vi "Dashboard Main.vi"() -> ()   [LabVIEW 2012]
uses:
  <vilib>/Utility/config.llb/Read Key (String).vi
  <vilib>/Utility/config.llb/Read Key (I32).vi
  <vilib>/Utility/config.llb/Write Key (String).vi
  <vilib>/Utility/config.llb/Write Key (I32).vi
  <vilib>/Utility/config.llb/NI_LVConfig.lvlib
panel:
  in  "Enable 4":bool
  in  "Camera Settings 2":T1={"Frate Rate"=30, "Compression"=30, "Size"=1} {"Frate Rate" scale=1.0..30.0; "Size" items=["640x480", "320x240", "160x120"]}
  in  "Enable 3":bool
  out "Mbps 3":dbl format="%#.1g"
  in  "Enable 2":bool
  in  "DB Camera Config 2":bool
  out "Mbps 2":bool
  out "fps 2":dbl format="%#.1g"
  out "Camera Image 2":T2(plugin-control)
  out "Battery Value":dbl(slide) scale=0.0..14.0 scale format="%#_2e"
  out "Battery":sgl(graph)
  in  "Camera Settings":T1={"Frate Rate"=30, "Compression"=30, "Size"=1} {"Frate Rate" scale=1.0..30.0; "Size" items=["640x480", "320x240", "160x120"]}
  out "Mode":T3(ring)=enum."Auto Disabled"
  out "JS1 Z":dbl(slide) scale=-1.0..1.0 scale format="%#_2e"
  out "JS2 Z":dbl(slide) scale=-1.0..1.0 scale format="%#_2e"
  out "Joystick 1":cluster{"X":dbl, "Y":dbl}[](graph)
  out "Joystick 2":cluster{"X":dbl, "Y":dbl}[](graph)
  out "JS Buttons 1":T4
  out "JS Buttons 2":T4
  out "MotorSlide4":dbl(slide) scale=-1.0..1.0 scale format="%#_2e"
  out "MotorSlide3":dbl(slide) scale=-1.0..1.0 scale format="%#_2e"
  out "MotorSlide2":dbl(slide) scale=-1.0..1.0 scale format="%#_2e"
  in  "MotorName3":string="Front Left"
  in  "MotorName4":string="Front Right"
  in  "MotorName1":string="Rear Left"
  in  "MotorName2":string="Rear Right"
  out "MotorChart4":dbl(graph)
  out "MotorChart3":dbl(graph)
  out "MotorChart2":dbl(graph)
  out "MotorSlide1":dbl(slide) scale=-1.0..1.0 scale format="%#_2e"
  out "MotorChart1":dbl(graph)
  out "Robot IP":string
  in  "Dashboard Tab":enum32{"Controls", "Test"}(tab)
  out "Climb Mode":bool
  out "Shooter Ready":bool
  out "Driver Ready":bool
  out "Manual Mode":bool
  in  "Slider":dbl(slide) scale=0.0..100.0 scale format="%#_3g"
  in  "On/Off":bool caption="Solenoid"
  in  "Test Name":u16(ring) items=["Select the test to run...", "Example Test", "-------------------------------", "List of tests is built in robot code.", "Replace with your own automated tests."]
  in  "Test Tree":string(tree)
  in  "Motor":cluster{"Value":dbl, "Enable":bool} {"Value" scale=-1.0..1.0 scale format="%#_3g"}
  out "Progress":T5 {"Test Progress" scale=0.0..100.0}
  in  "Rev/Fwd":cluster{"Forward":bool, "Reverse":bool}
  in  "Ring":u16(ring) items=["Auto", "Fixed indoor", "Fixed outdoor 1", "Fixed outdoor 2", "Fixed fluorescent 1", "Fixed fluorescent 2", "Hold current"]
  in  "Viewer":enum32{"Camera Image", "Variables"}(tab)
  out "Mbps":dbl format="%#.1g"
  in  "Enable":bool
  in  "DB Camera Config":bool
  out "Mbps":bool
  out "fps":dbl format="%#.1g"
  out "Image Error Message":string="Timeout in Camera Communications"
  out "Camera Image":T2(plugin-control)
  out "Tree":string(tree)
  # "Drive & Motors"
  # "Robot IP:"
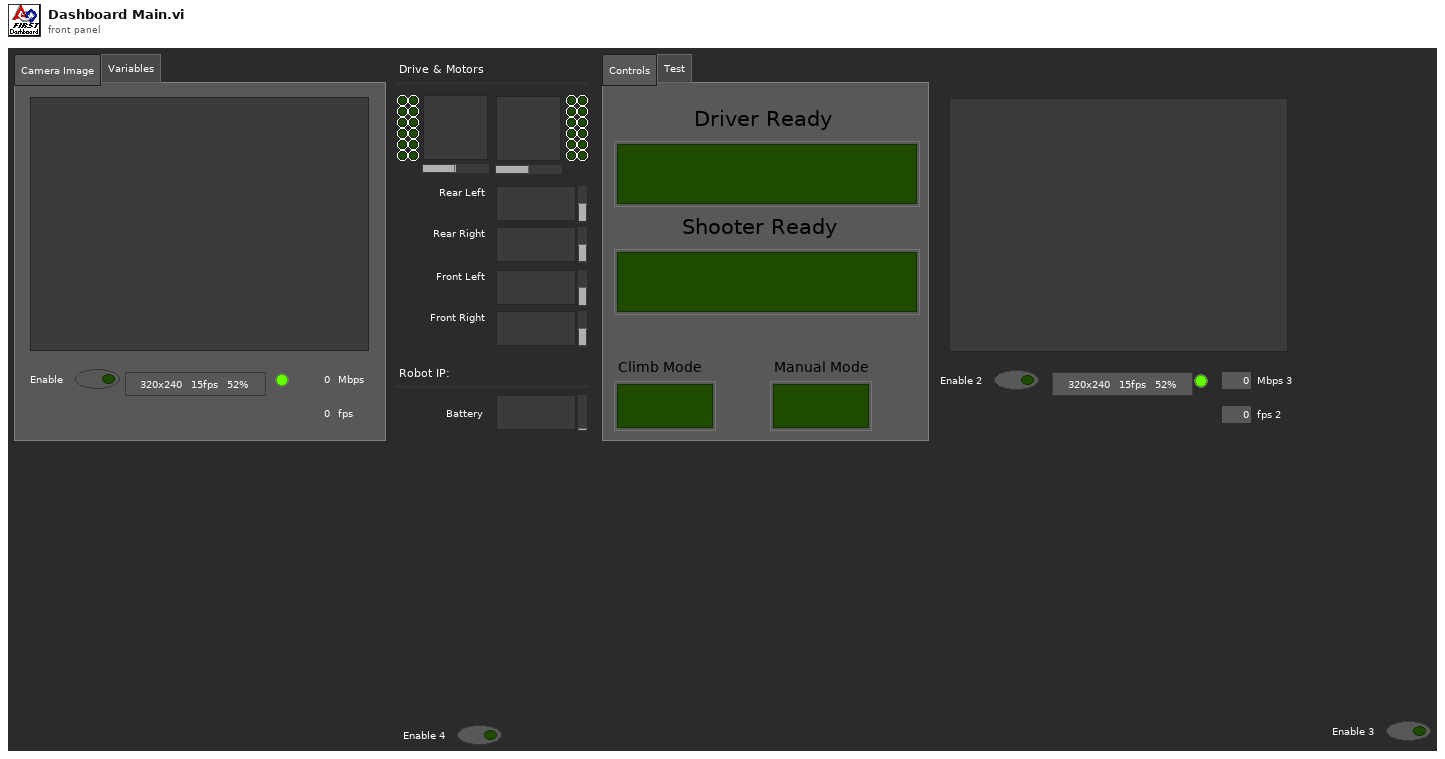
[diagram p1: front panel]
types:
  T1 = cluster{"Frate Rate":i32, "Compression":i32, "Size":u16}
  T2 = typedef "IMAQ Image.ctl" = refnum<image>
  T3 = enum8{"Tele-Op Disabled", "Tele-Op Enabled", "Auto Disabled", "Auto Enabled", "Test Disabled", "Test Enabled", ""}
  T4 = cluster{bool, bool, bool, bool, bool, bool, bool, bool, bool, bool, bool, bool}
  T5 = cluster{"Test Progress":u8, "Test Progress Text":string}
  T6 = typedef "Image Type" = u32
  T7 = typedef "NI_LVConfig.lvlib/Config Data RefNum.ctl" = refnum<k1>
  T8 = cluster{"Competition mode":bool, "Robot Link":bool, "Autonomous":bool, "Enabled":bool, "E-Stop":bool, "Simulated":bool, "TestMode":bool, "Docked Window":bool}
  T9 = cluster{"Boolean Array[0]":bool, "Boolean Array[1]":bool, "Boolean Array[2]":bool, "Boolean Array[3]":bool, "Boolean Array[4]":bool, "Boolean Array[5]":bool, "Boolean Array[6]":bool, "Boolean Array[7]":bool, "Boolean Array[8]":bool, "Boolean Array[9]":bool, "Boolean Array[10]":bool, "Boolean Array[11]":bool}
  T10 = typedef "LVRectTypeDef.ctl" = cluster{"Left":i16, "Top":i16, "Right":i16, "Bottom":i16}
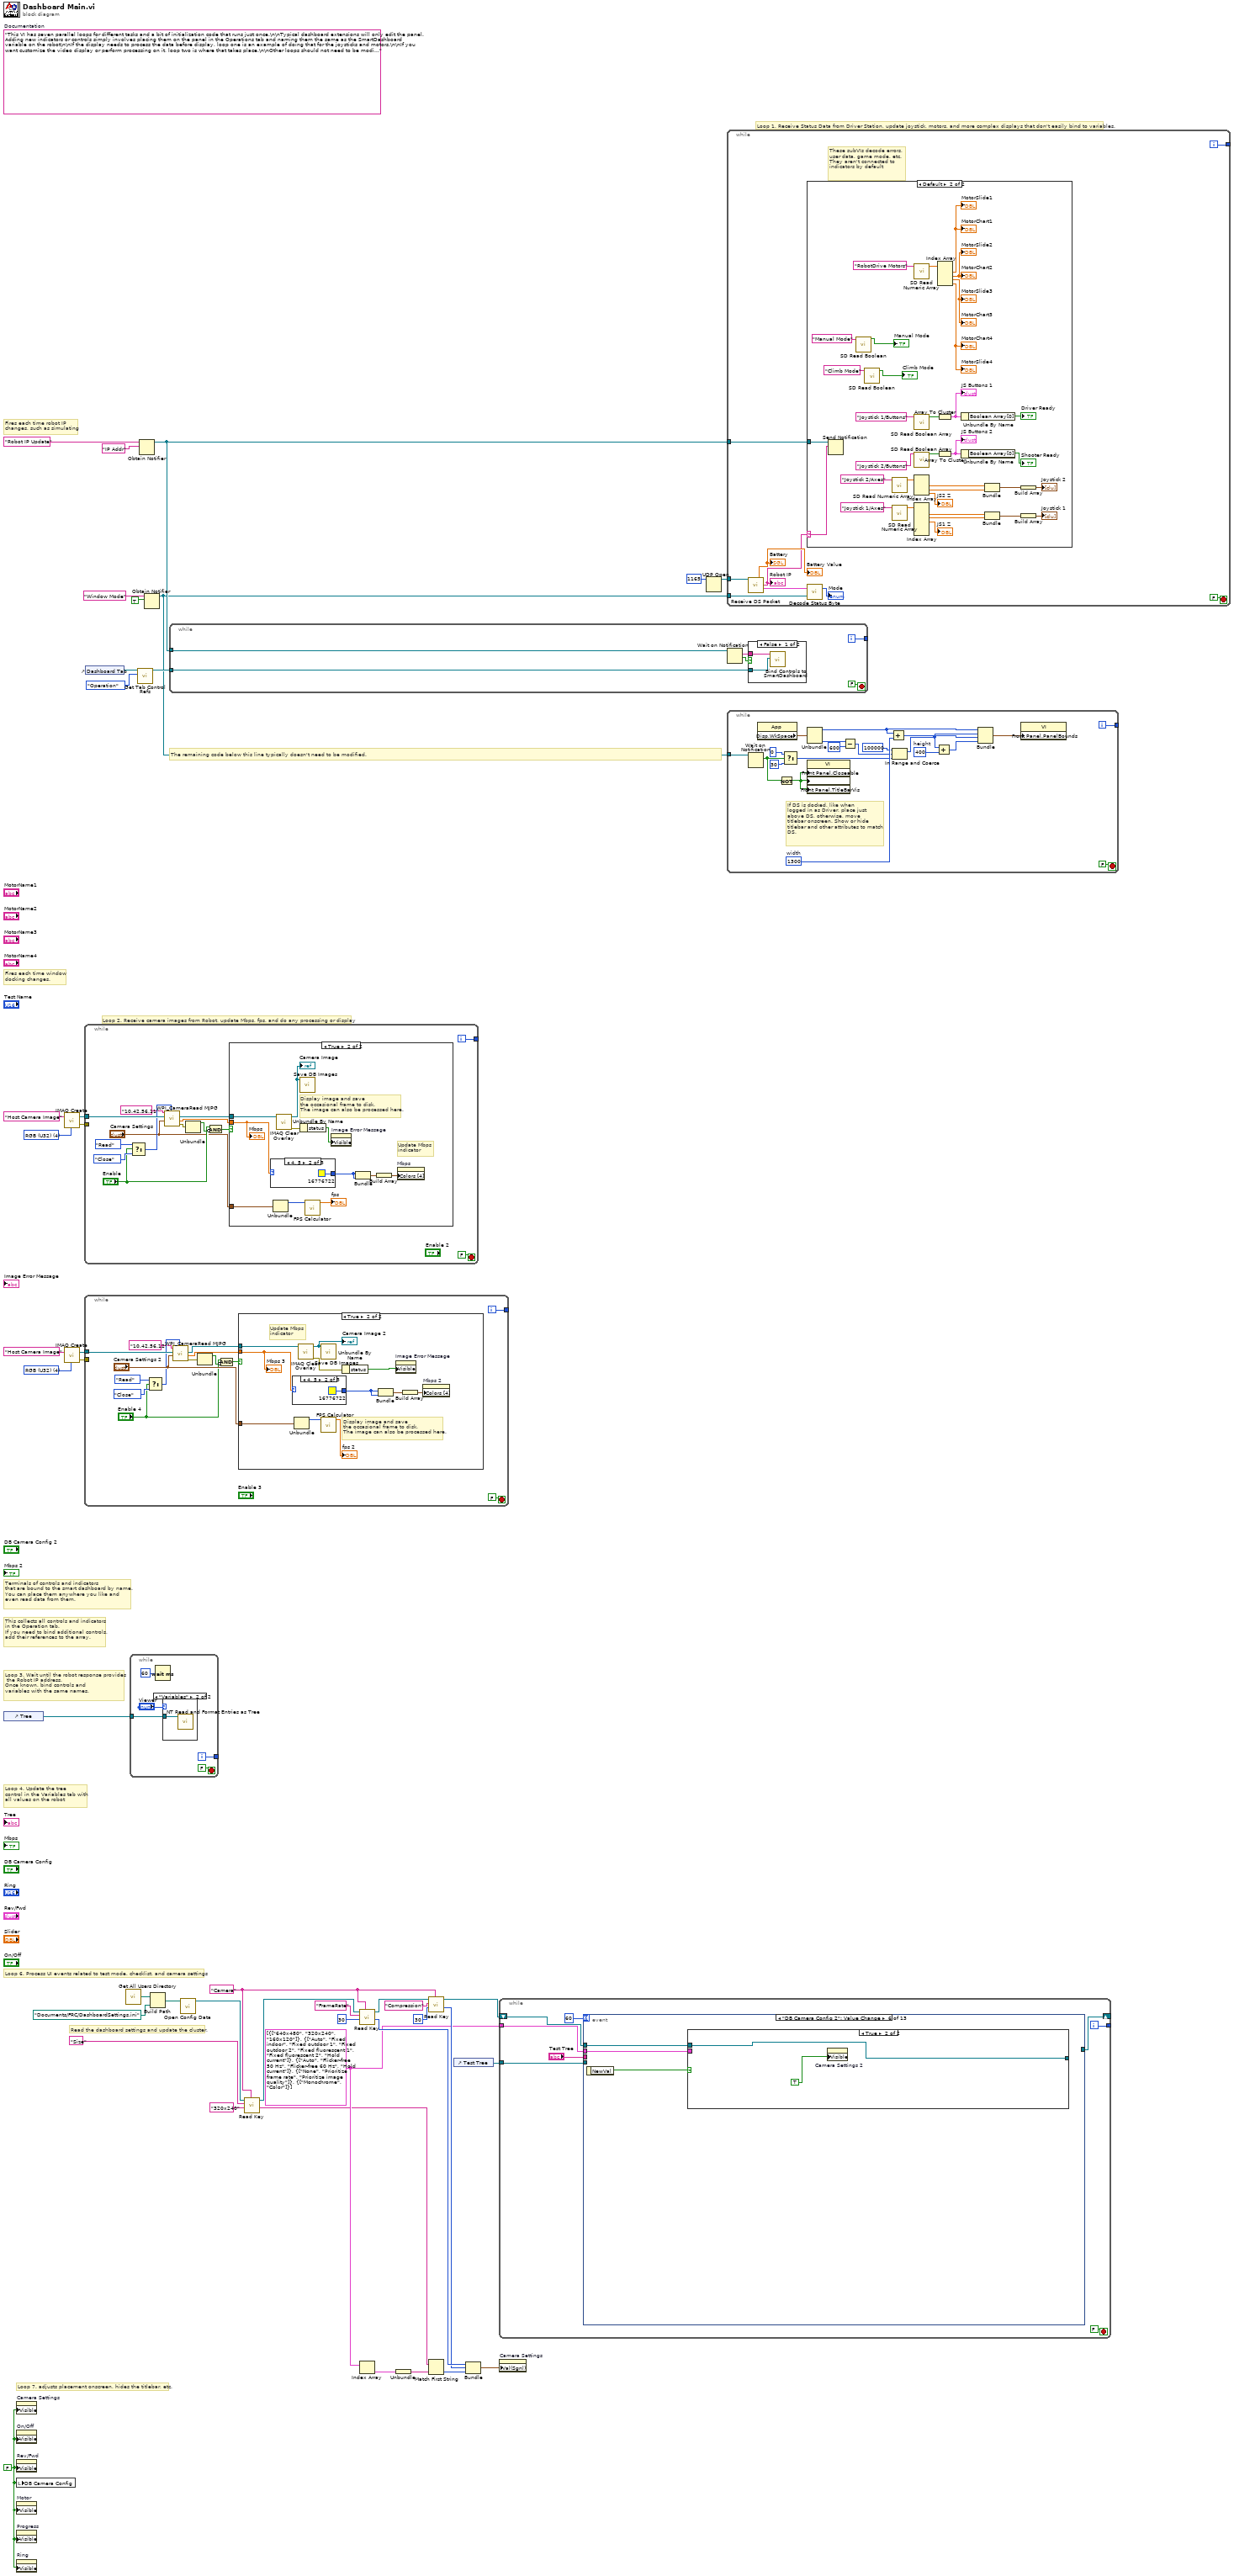
[diagram p0: block diagram]
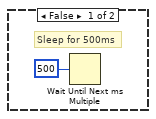
[diagram p2: hidden frame]
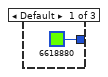
[diagram p3: hidden frame]
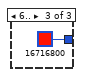
[diagram p4: hidden frame]
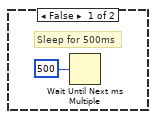
[diagram p6: hidden frame]
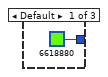
[diagram p7: hidden frame]
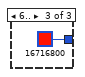
[diagram p8: hidden frame]
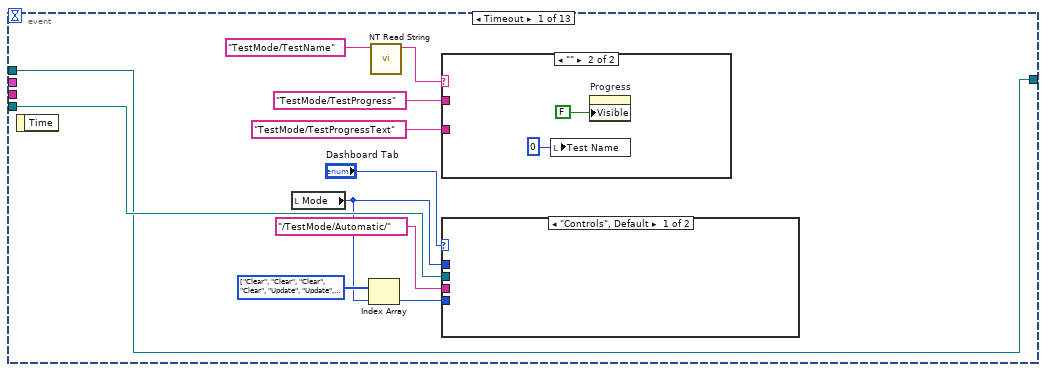
[diagram p9: hidden frame]
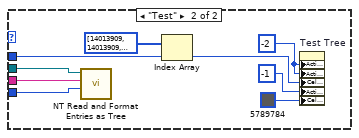
[diagram p10: hidden frame]
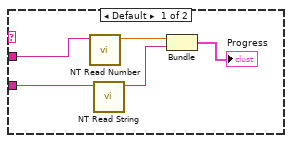
[diagram p11: hidden frame]
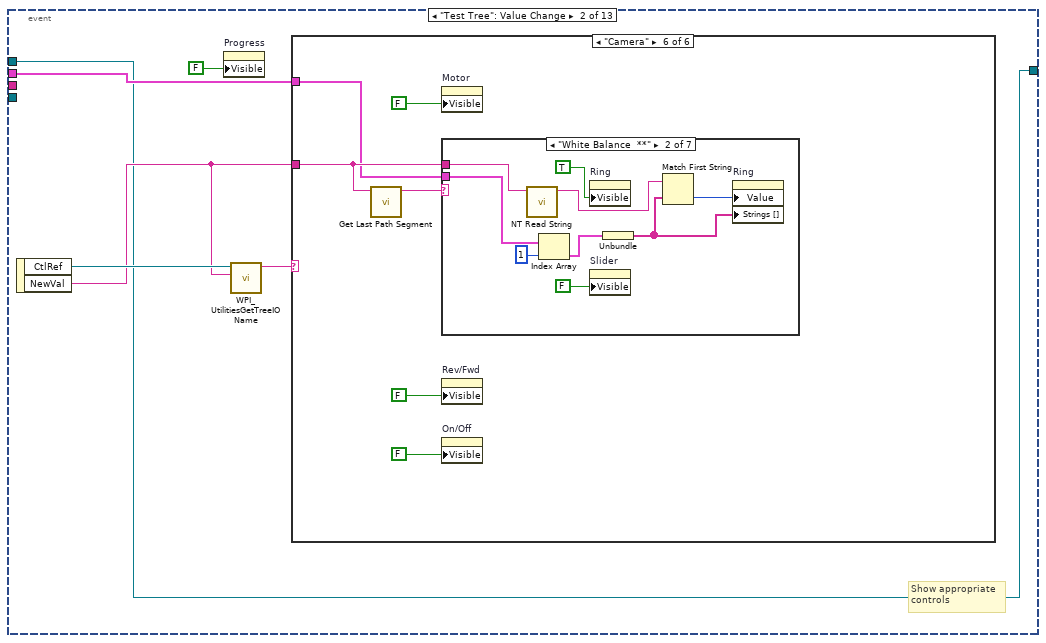
[diagram p12: hidden frame]
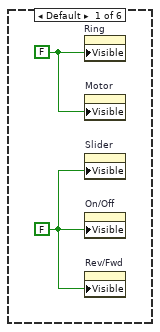
[diagram p13: hidden frame]
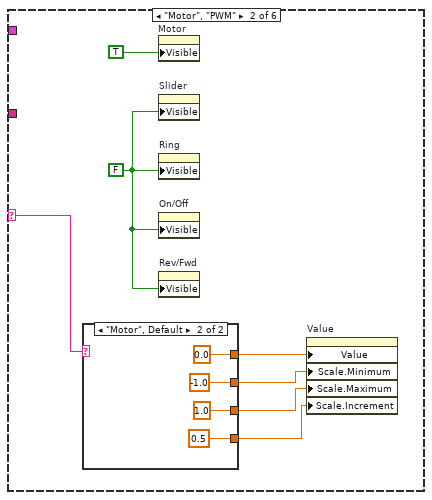
[diagram p14: hidden frame]
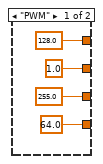
[diagram p15: hidden frame]
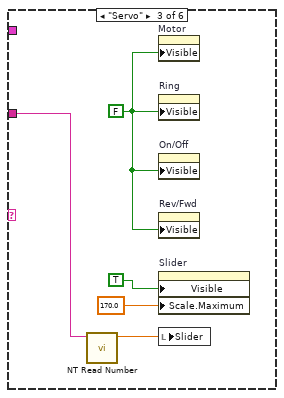
[diagram p16: hidden frame]
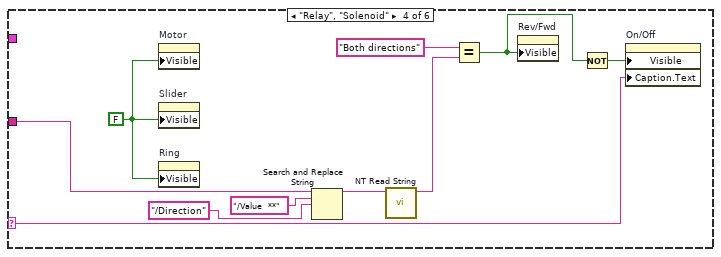
[diagram p17: hidden frame]
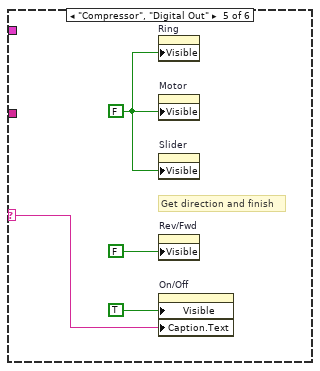
[diagram p18: hidden frame]
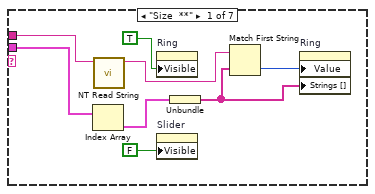
[diagram p19: hidden frame]
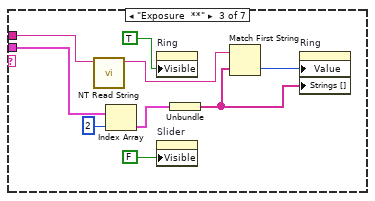
[diagram p20: hidden frame]
diagram:
  w4 = T6 4 items=["Grayscale (U8)", "Grayscale (I16)", "Grayscale (SGL)", "Complex (CSG)", "RGB (U32)", "HSL (U32)", "RGB (U64)"] ("Image Type")
  w23 = "Camera"
  w15 = cluster{string[]}[] [{["640x480", "320x240", "160x120"]}, {["Auto", "Fixed indoor", "Fixed outdoor 1", "Fixed outdoor 2", "Fixed fluorescent 1", "Fixed fluorescent 2", "Hold current"]}, {["Auto", "Flicker-free 50 Hz", "Flicker-free 60 Hz", "Hold current"]}, {["None", "Prioritize frame rate", "Prioritize image quality"]}, {["Monochrome", "Color"]}]
  w29 = FALSE ("Visible")
  (unwired) "This VI has seven parallel loops for different tasks and a bit of initialization code that runs just once.\n\nTypical dashboard extensions will only edit the panel. Adding new indicators or controls simply involves placing them on the panel in the Operations tab and naming them the same as the SmartDashboard variable on the robot\n\nIf the display needs to process the data before display, loop one is an example of doing that for the joysticks and motors.\n\nIf you want customize the video display or perform processing on it, loop two is where that takes place.\n\nOther loops should not need to be modified. They are pretty standard, and document the task they perform."  # Documentation
  w42 = T6 4 items=["Grayscale (U8)", "Grayscale (I16)", "Grayscale (SGL)", "Complex (CSG)", "RGB (U32)", "HSL (U32)", "RGB (U64)"] ("Image Type")
  # "Fires each time robot IP\nchanges, such as simulating"
  # "Fires each time window\ndocking changes."
  # "This collects all controls and indicators\nin the Operation tab.\nIf you need to bind additional controls,\nadd their references to the array."
  # "The remaining code below this line typically doesn't need to be modified."
  # "Loop 6. Process UI events related to test mode, checklist, and camera settings"
  # "Read the dashboard settings and update the cluster."
  # "Terminals of controls and indicators\nthat are bound to the smart dashboard by name.\nYou can place them anywhere you like and\neven read data from them."
  # "Loop 4. Update the tree\ncontrol in the Variables tab with\nall values on the robot"
  # "Loop 3. Wait until the robot response provides\n the Robot IP address.\nOnce known, bind controls and\nvariables with the same names."
  # "Loop 7. adjusts placement onscreen, hides the titlebar, etc."
  # "Loop 1. Receive Status Data from Driver Station, update joystick, motors, and more complex displays that don't easily bind to variables."
  # "Loop 2. Receive camera images from Robot, update Mbps, fps, and do any processing or display"
  n1 = control-ref of="Tree"() -> (w6:refnum<vi>)
  n2 = property on="Camera Settings" class="Clust (strict)"("Visible"=w29) -> ()  [unwired: 2 in, 2 out]
  n3 = property on="On/Off" class="Bool (strict)"("Visible"=w29) -> ()  [unwired: 2 in, 2 out]
  n4 = property on="Rev/Fwd" class="Clust (strict)"("Visible"=w29) -> ()  [unwired: 2 in, 2 out]
  n5 = local write "DB Camera Config"(w29) -> ()
  n6 = property on="Motor" class="Clust (strict)"("Visible"=w29) -> ()  [unwired: 2 in, 2 out]
  n7 = property on="Progress" class="Clust (strict)"("Visible"=w29) -> ()  [unwired: 2 in, 2 out]
  n8 = property on="Ring" class="Ring (strict)"("Visible"=w29) -> ()  [unwired: 2 in, 2 out]
  n9 = call "IMAQ Create"("Image Name"="Host Camera Image", "Image Type"=w42) -> ("New Image"=w40:T2, "error out"=w39:errorcluster)  [unwired: 2 in, 1 out]
  n10 = call "IMAQ Create"("Image Name"="Host Camera Image", "Image Type"=w4) -> ("New Image"=w2:T2, "error out"=w1:errorcluster)  [unwired: 2 in, 1 out]
  n11 = while {
    tunnel: w40 -> [w56]
    tunnel: w39 -> [_]
    tunnel: [w57] -> _
    i -> [w57]
    stop <- FALSE stop-if-true
    n12 = Select(t=enum16{"Read", "Reopen", "Close"}."Read" ("Operation"), s="Enable", f=enum16{"Read", "Reopen", "Close"}."Close" ("Operation")) -> (s? t:f=w51:enum16{"Read", "Reopen", "Close"})
    n13 = call <vilib>:"WPI_CameraRead MJPG.vi"("Operation"=w51, "Camera Settings"="Camera Settings", "Image"=w56, "address"="10.42.56.11") -> ("error out"=w50:errorcluster, "Bandwidth (kbps)"=w54:dbl, "Image Out"=w55:T2)  [unwired: 5 in]
    n14 = Unbundle(w50) -> ("status"=w48:bool)  [unwired: 2 out]
    n15 = Compound Arithmetic op=AND("Enable", invert w48) -> (w47:bool)
    n16 = case shown="True" w47 {
      tunnel: "Camera Settings" -> [_ w61]
      tunnel: w55 -> [_ w64]
      tunnel: w54 -> [_ w63]
      frame False {
        # "Sleep for 500ms"
        n17 = Wait Until Next ms Multiple(millisecond multiple=u32 500) -> ()  [unwired: 1 out]
      }
      frame True {
        # "Display image and save\nthe occasional frame to disk.\nThe image can also be processed here."
        # "Update Mbps\nindicator"
        n18 = case shown="4, 5" w63 {
          tunnel: [u32 6618880 ("Color Box") u32 16776722 ("Color Box") u32 16716800 ("Color Box")] -> w65
          frame Default {
          }
          frame 4, 5 {
          }
          frame 6.. {
          }
        }
        n19 = Unbundle(w61) -> ("Frate Rate"=w60:i32)  [unwired: 2 out]
        n20 = call "IMAQ Clear Overlay"("Image"=w64) -> ("error out"=w69:errorcluster, "Image Out"=w68:T2)  [unwired: 2 in, 7 out]
        "Camera Image" <- w68
        n21 = call "Save DB Images.vi"("Image"=w68) -> ()  [unwired: 2 in, 1 out]
        n22 = Unbundle By Name(w69) -> ("status"=w70:bool)
        n23 = call "FPS Calculator.vi"("Average Count"=w60) -> ("fps"=→"fps":dbl)  [unwired: 10 in]
        n24 = property on="Image Error Message" class="Str"("Visible"=w70) -> ()  [unwired: 2 in, 2 out]
        n25 = Bundle("Color Box"=w65, "Color Box"=w65) -> (w67:cluster{"Color Box":u32, "Color Box":u32})  [unwired: 1 out]
        n26 = Build Array(w67) -> (w66:cluster{"Color Box":u32, "Color Box":u32}[])
        n27 = property on="Mbps" class="Bool (strict)"("Colors [4]"=w66) -> ()  [unwired: 2 in, 2 out]
        "Mbps" <- w63
      }
    }
  }
  n28 = while {
    tunnel: w2 -> [w84]
    tunnel: w1 -> [_]
    tunnel: [w86] -> _
    i -> [w86]
    stop <- FALSE stop-if-true
    n29 = Select(t=enum16{"Read", "Reopen", "Close"}."Read" ("Operation"), s="Enable 4", f=enum16{"Read", "Reopen", "Close"}."Close" ("Operation")) -> (s? t:f=w79:enum16{"Read", "Reopen", "Close"})
    n30 = call <vilib>:"WPI_CameraRead MJPG.vi"("Operation"=w79, "Camera Settings"="Camera Settings 2", "Image"=w84, "address"="10.42.56.12") -> ("error out"=w78:errorcluster, "Bandwidth (kbps)"=w82:dbl, "Image Out"=w83:T2)  [unwired: 5 in]
    n31 = Unbundle(w78) -> ("status"=w76:bool)  [unwired: 2 out]
    n32 = Compound Arithmetic op=AND("Enable 4", invert w76) -> (w75:bool)
    n33 = case shown="True" w75 {
      tunnel: "Camera Settings 2" -> [_ w94]
      tunnel: w83 -> [_ w95]
      tunnel: w82 -> [_ w90]
      frame False {
        # "Sleep for 500ms"
        n34 = Wait Until Next ms Multiple(millisecond multiple=u32 500) -> ()  [unwired: 1 out]
      }
      frame True {
        # "Display image and save\nthe occasional frame to disk.\nThe image can also be processed here."
        # "Update Mbps\nindicator"
        n35 = case shown="4, 5" w90 {
          tunnel: [u32 6618880 ("Color Box") u32 16776722 ("Color Box") u32 16716800 ("Color Box")] -> w96
          frame Default {
          }
          frame 4, 5 {
          }
          frame 6.. {
          }
        }
        n36 = Unbundle(w94) -> ("Frate Rate"=w93:i32)  [unwired: 2 out]
        n37 = call "IMAQ Clear Overlay"("Image"=w95) -> ("error out"=w99:errorcluster, "Image Out"=w92:T2)  [unwired: 2 in, 7 out]
        "Camera Image 2" <- w92
        n38 = call "Save DB Images.vi"("Image"=w92) -> ()  [unwired: 2 in, 1 out]
        n39 = call "FPS Calculator.vi"("Average Count"=w93) -> ("fps"=→"fps 2":dbl)  [unwired: 10 in]
        n40 = Unbundle By Name(w99) -> ("status"=w89:bool)
        n41 = Bundle("Color Box"=w96, "Color Box"=w96) -> (w98:cluster{"Color Box":u32, "Color Box":u32})  [unwired: 1 out]
        n42 = property on="Image Error Message" class="Str"("Visible"=w89) -> ()  [unwired: 2 in, 2 out]
        n43 = Build Array(w98) -> (w97:cluster{"Color Box":u32, "Color Box":u32}[])
        n44 = property on="Mbps 2" class="Bool (strict)"("Colors [4]"=w97) -> ()  [unwired: 2 in, 2 out]
        "Mbps 3" <- w90
      }
    }
  }
  n45 = control-ref of="Dashboard Tab"() -> (w37:refnum<vi>)
  n46 = call "Get All Users Directory.vi"() -> ("All User Path"=w28:path)
  n47 = while {
    tunnel: [w104] -> _
    tunnel: w6 -> [w103]
    i -> [w104]
    stop <- FALSE stop-if-true
    n48 = Wait (ms)(milliseconds to wait=u32 60) -> ()  [unwired: 1 out]
    n49 = case shown="\"Variables\"" "Viewer" {
      tunnel: w103 -> [_ w108]
      frame Default {
      }
      frame "Variables" {
        n50 = call <vilib>:"NT Read and Format Entries as Tree.vi"("Tree Refnum"=w108) -> ()  [unwired: 9 in, 2 out]
      }
    }
  }
  n51 = call <vilib>:"Get Tab Control Refs.vi"("Page Index"=enum32{"Operation", "Test"}."Operation" ("Dashboard Tab"), "TabControl in"=w37) -> ("ControlsOnPage"=w38:refnum<vi>[])  [unwired: 9 in]
  n52 = Obtain Notifier(name (unnamed)="Robot IP Update", notification data type="IP Addr" ("name (unnamed)")) -> (notifier out=w34:refnum<notifier>)  [unwired: 2 in, 2 out]
  n53 = Obtain Notifier(name (unnamed)="Window Mode", notification data type=TRUE) -> (notifier out=w30:refnum<notifier>)  [unwired: 2 in, 2 out]
  n54 = Build Path(base path=w28, name or relative path=path "Documents/FRC/DashboardSettings.ini") -> (appended path=w27:path)
  n55 = while {
    tunnel: w38 -> [w114]
    tunnel: w34 -> [w111]
    tunnel: [w109] -> _
    i -> [w109]
    stop <- FALSE stop-if-true
    n56 = Wait on Notification(notifier=w111) -> (notification=w110:string, timed out?=w112:bool)  [unwired: 3 in, 2 out]
    n57 = case shown="False" w112 {
      tunnel: w114 -> [w116 _]
      tunnel: w110 -> [w115 _]
      frame False {
        n58 = call <vilib>:"Bind Controls to SmartDashboard.vi"("Bound Control Refs"=w116, "Server IP Address"=w115) -> ()  [unwired: 10 in]
      }
      frame True {
      }
    }
  }
  n59 = call <vilib>:"Open Config Data.vi"("configuration file path"=w27) -> ("refnum"=w26:T7)  [unwired: 8 in, 2 out]
  n60 = call-poly <vilib>:"Read Key.vi"("section"=w23, "default value"="320x240", "key"="Size", "refnum"=w26) -> ("value"=w13:string, "refnum out"=w10:T7)  [unwired: 2 in, 4 out]
  n61 = call-poly <vilib>:"Read Key.vi"("section"=w23, "default value"=30, "key"="FrameRate", "refnum"=w10) -> ("value"=w18:i32, "refnum out"=w9:T7)  [unwired: 1 in, 5 out]
  n62 = Index Array(array=w15) -> (element=w16:cluster{string[]})  [unwired: 1 in]
  n63 = Unbundle(w16) -> (w14:string[])
  n64 = call-poly <vilib>:"Read Key.vi"("section"=w23, "default value"=30, "key"="Compression", "refnum"=w9) -> ("value"=w17:i32, "refnum out"=w7:T7)  [unwired: 1 in, 5 out]
  n65 = Match First String(2:w14, 3:w13) -> (0:w12:i32)  [unwired: 1 out]
  n66 = control-ref of="Test Tree"() -> (w5:refnum<vi>)
  n67 = Bundle("value"=w18, "value"=w17, "index"=w12) -> (w8:cluster{"value":i32, "value":i32, "index":i32})  [unwired: 1 out]
  n68 = while {
    tunnel: w15 -> [w121]
    shift-right: [w120] -> _
    shift-left: w7 -> [w119]
    tunnel: [w118] -> _
    tunnel: w5 -> [w117]
    i -> [w118]
    stop <- FALSE stop-if-true
    n69 = event shown="[5] \"DB Camera Config 2\": Value Change" {
      selector: _ -> [_ _ _ _ _ _ _ _ _ _ _ _ _]
      dyn-events: _ -> [_ _ _ _ _ _ _ _ _ _ _ _ _]
      timeout: u32 60 ("milliseconds to wait") -> [_ _ _ _ _ _ _ _ _ _ _ _ _]
      tunnel: w117 -> [w131 _ _ _ _ _ _ _ _ _ _ _ _]
      tunnel: "Test Tree" -> [_ _ _ _ _ _ _ _ w337 w345 w347 w351 w359]
      tunnel: w121 -> [_ w153 _ _ w265 w289 w319 w331 _ _ _ _ _]
      tunnel: [w125 w152 _ w255 w264 _ w312 w324 w336 w343 w346 w350 w358] -> w120
      tunnel: w119 -> [w125 w152 _ w255 w263 w288 w312 w324 w336 w343 w346 w350 w358]
      event Timeout {
        w130 = enum16{"Update", "Clear"}[] [enum."Clear", enum."Clear", enum."Clear", enum."Clear", enum."Update", enum."Update", enum."Clear"] items=["Update", "Clear"]
        n70 = event-data() -> ()  [unwired: 1 in, 1 out]
        n71 = local read "Mode"() -> (w128:T3)
        n72 = Index Array(array=w130, index=w128) -> (element=w129:enum16{"Update", "Clear"})
        n73 = call <vilib>:"NT Read String.vi"("Name"="TestMode/TestName") -> ("String"=w134:string)  [unwired: 9 in, 1 out]
        n74 = case shown="\"\"" w134 {
          tunnel: "TestMode/TestProgress" ("Name") -> [w146 _]
          tunnel: "TestMode/TestProgressText" ("Name") -> [w145 _]
          frame Default {
            n75 = call <vilib>:"NT Read Number.vi"("Name"=w146) -> ("Numeric"=w147:dbl)  [unwired: 9 in, 1 out]
            n76 = call <vilib>:"NT Read String.vi"("Name"=w145) -> ("String"=w148:string)  [unwired: 9 in, 1 out]
            n77 = Bundle("Numeric"=w147, "String"=w148) -> (→"Progress":cluster{"Numeric":dbl, "String":string})  [unwired: 1 in]
          }
          frame "" {
            n78 = local write "Test Name"(u16 0) -> ()
            n79 = property on="Progress" class="Clust (strict)"("Visible"=FALSE) -> ()  [unwired: 2 in, 2 out]
          }
        }
        n80 = case shown="\"Controls\", Default" "Dashboard Tab" {
          tunnel: w131 -> [_ w144]
          tunnel: "/TestMode/Automatic/" ("Name Pattern") -> [_ w143]
          tunnel: w129 -> [_ w142]
          tunnel: w128 -> [_ w140]
          frame "Controls", Default {
          }
          frame "Test" {
            w139 = -2 ("Active Item:Row Number")
            n81 = call <vilib>:"NT Read and Format Entries as Tree.vi"("Operation"=w142, "Name Pattern"=w143, "Tree Refnum"=w144) -> ()  [unwired: 7 in, 2 out]
            n82 = Index Array(array=u32[] [14013909, 14013909, 14013909, 14013909, 14013909, 16777215, 14013909], index=w140) -> (element=w138:u32)
            n83 = property on="Test Tree" class="Tree (strict)"("Active Item Row Number"=w139, "ActiveColNum"=w139, "CellBG"=w138, "Active Item Row Number"=-1 ("Active Item:Row Number"), "CellBG"=u32 5789784 ("Color Box")) -> ()  [unwired: 2 in, 2 out]
          }
        }
      }
      event "Test Tree": Value Change {
        # "Show appropriate\ncontrols"
        n84 = event-data() -> ("CtlRef"=w156:refnum<vi>, "NewVal"=w154:string)  [unwired: 1 in]
        n85 = property on="Progress" class="Clust (strict)"("Visible"=FALSE) -> ()  [unwired: 2 in, 2 out]
        n86 = call <vilib>:"WPI_UtilitiesGetTreeIOName.vi"("NewVal"=w154, "TreeControl in"=w156) -> ("I/O Name"=w157:string)  [unwired: 9 in]
        n87 = case shown="\"Camera\"" w157 {
          selector: w157 -> [_ w164 _ w182 w191 _]
          tunnel: w154 -> [_ _ w179 w181 _ w198]
          tunnel: w153 -> [_ _ _ _ _ w197]
          frame Default {
            w159 = FALSE ("Visible")
            w158 = FALSE ("Visible")
            n88 = property on="Ring" class="Ring (strict)"("Visible"=w158) -> ()  [unwired: 2 in, 2 out]
            n89 = property on="Motor" class="Clust (strict)"("Visible"=w158) -> ()  [unwired: 2 in, 2 out]
            n90 = property on="Slider" class="Slide (strict)"("Visible"=w159) -> ()  [unwired: 2 in, 2 out]
            n91 = property on="On/Off" class="Bool (strict)"("Visible"=w159) -> ()  [unwired: 2 in, 2 out]
            n92 = property on="Rev/Fwd" class="Clust (strict)"("Visible"=w159) -> ()  [unwired: 2 in, 2 out]
          }
          frame "Motor", "PWM" {
            w165 = FALSE ("Visible")
            n93 = case shown="\"Motor\", Default" w164 {
              tunnel: [1.0 ("Value") -1.0 ("Value")] -> w163
              tunnel: [255.0 ("Value") 1.0 ("Value")] -> w162
              tunnel: [128.0 ("Value") 0.0 ("Value")] -> w161
              tunnel: [64.0 ("Value") 0.5 ("Value")] -> w160
              frame "PWM" {
              }
              frame "Motor", Default {
              }
            }
            n94 = property on="Motor" class="Clust (strict)"("Visible"=TRUE) -> ()  [unwired: 2 in, 2 out]
            n95 = property on="Slider" class="Slide (strict)"("Visible"=w165) -> ()  [unwired: 2 in, 2 out]
            n96 = property on="Ring" class="Ring (strict)"("Visible"=w165) -> ()  [unwired: 2 in, 2 out]
            n97 = property on="On/Off" class="Bool (strict)"("Visible"=w165) -> ()  [unwired: 2 in, 2 out]
            n98 = property on="Rev/Fwd" class="Clust (strict)"("Visible"=w165) -> ()  [unwired: 2 in, 2 out]
            n99 = property on="Value" class="Slide (strict)"("Value"=w161, "Scale.Minimum"=w163, "Scale.Maximum"=w162, "Scale.Increment"=w160) -> ()  [unwired: 2 in, 2 out]
          }
          frame "Servo" {
            w177 = FALSE ("Visible")
            n100 = call <vilib>:"NT Read Number.vi"("Name"=w179) -> ("Numeric"=w178:dbl)  [unwired: 9 in, 1 out]
            n101 = property on="Motor" class="Clust (strict)"("Visible"=w177) -> ()  [unwired: 2 in, 2 out]
            n102 = property on="Ring" class="Ring (strict)"("Visible"=w177) -> ()  [unwired: 2 in, 2 out]
            n103 = property on="On/Off" class="Bool (strict)"("Visible"=w177) -> ()  [unwired: 2 in, 2 out]
            n104 = property on="Rev/Fwd" class="Clust (strict)"("Visible"=w177) -> ()  [unwired: 2 in, 2 out]
            n105 = property on="Slider" class="Slide (strict)"("Visible"=TRUE, "Scale.Maximum"=170.0 ("Scale.Range:Maximum")) -> ()  [unwired: 2 in, 2 out]
            n106 = local write "Slider"(w178) -> ()
          }
          frame "Relay", "Solenoid" {
            w180 = FALSE ("Visible")
            n107 = property on="Motor" class="Clust (strict)"("Visible"=w180) -> ()  [unwired: 2 in, 2 out]
            n108 = property on="Slider" class="Slide (strict)"("Visible"=w180) -> ()  [unwired: 2 in, 2 out]
            n109 = property on="Ring" class="Ring (strict)"("Visible"=w180) -> ()  [unwired: 2 in, 2 out]
            n110 = Search and Replace String(input string=w181, search string="/Value  **", replace string="/Direction") -> (result string=w187:string)  [unwired: 5 in, 3 out]
            n111 = call <vilib>:"NT Read String.vi"("Name"=w187) -> ("String"=w185:string)  [unwired: 9 in, 1 out]
            n112 = Equal?(x="Both directions", y=w185) -> (x = y?=w183:bool)
            n113 = property on="Rev/Fwd" class="Clust (strict)"("Visible"=w183) -> ()  [unwired: 2 in, 2 out]
            n114 = Not(x=w183) -> (.not. x?=w184:bool)
            n115 = property on="On/Off" class="Bool (strict)"("Visible"=w184, "Caption.Text"=w182) -> ()  [unwired: 2 in, 2 out]
          }
          frame "Compressor", "Digital Out" {
            w190 = FALSE ("Visible")
            # "Get direction and finish"
            n116 = property on="Ring" class="Ring (strict)"("Visible"=w190) -> ()  [unwired: 2 in, 2 out]
            n117 = property on="Motor" class="Clust (strict)"("Visible"=w190) -> ()  [unwired: 2 in, 2 out]
            n118 = property on="Slider" class="Slide (strict)"("Visible"=w190) -> ()  [unwired: 2 in, 2 out]
            n119 = property on="Rev/Fwd" class="Clust (strict)"("Visible"=FALSE) -> ()  [unwired: 2 in, 2 out]
            n120 = property on="On/Off" class="Bool (strict)"("Visible"=TRUE, "Caption.Text"=w191) -> ()  [unwired: 2 in, 2 out]
          }
          frame "Camera" {
            n121 = call <vilib>:"Get Last Path Segment.vi"("String in"=w198) -> ("String out"=w199:string)  [unwired: 10 in]
            n122 = property on="Motor" class="Clust (strict)"("Visible"=FALSE) -> ()  [unwired: 2 in, 2 out]
            n123 = case shown="\"White Balance  **\"" w199 {
              tunnel: w198 -> [w205 w214 w223 w232 w241 _ w247]
              tunnel: w197 -> [w203 w211 w220 w229 w238 _ _]
              frame "Size  **" {
                n124 = Index Array(array=w203) -> (element=w202:cluster{string[]})  [unwired: 1 in]
                n125 = call <vilib>:"NT Read String.vi"("Name"=w205) -> ("String"=w204:string)  [unwired: 9 in, 1 out]
                n126 = property on="Ring" class="Ring (strict)"("Visible"=TRUE) -> ()  [unwired: 2 in, 2 out]
                n127 = property on="Slider" class="Slide (strict)"("Visible"=FALSE) -> ()  [unwired: 2 in, 2 out]
                n128 = Unbundle(w202) -> (w200:string[])
                n129 = Match First String(2:w200, 3:w204) -> (0:w201:i32)  [unwired: 1 out]
                n130 = property on="Ring" class="Ring (strict)"("Value"=w201, "Strings []"=w200) -> ()  [unwired: 2 in, 2 out]
              }
              frame "White Balance  **" {
                n131 = call <vilib>:"NT Read String.vi"("Name"=w214) -> ("String"=w213:string)  [unwired: 9 in, 1 out]
                n132 = Index Array(array=w211, index=1) -> (element=w212:cluster{string[]})
                n133 = property on="Ring" class="Ring (strict)"("Visible"=TRUE) -> ()  [unwired: 2 in, 2 out]
                n134 = property on="Slider" class="Slide (strict)"("Visible"=FALSE) -> ()  [unwired: 2 in, 2 out]
                n135 = Unbundle(w212) -> (w209:string[])
                n136 = Match First String(2:w209, 3:w213) -> (0:w208:i32)  [unwired: 1 out]
                n137 = property on="Ring" class="Ring (strict)"("Value"=w208, "Strings []"=w209) -> ()  [unwired: 2 in, 2 out]
              }
              frame "Exposure  **" {
                n138 = call <vilib>:"NT Read String.vi"("Name"=w223) -> ("String"=w222:string)  [unwired: 9 in, 1 out]
                n139 = Index Array(array=w220, index=2) -> (element=w221:cluster{string[]})
                n140 = property on="Ring" class="Ring (strict)"("Visible"=TRUE) -> ()  [unwired: 2 in, 2 out]
                n141 = property on="Slider" class="Slide (strict)"("Visible"=FALSE) -> ()  [unwired: 2 in, 2 out]
                n142 = Unbundle(w221) -> (w217:string[])
                n143 = Match First String(2:w217, 3:w222) -> (0:w218:i32)  [unwired: 1 out]
                n144 = property on="Ring" class="Ring (strict)"("Value"=w218, "Strings []"=w217) -> ()  [unwired: 2 in, 2 out]
              }
              frame "Exposure Priority  **" {
                n145 = call <vilib>:"NT Read String.vi"("Name"=w232) -> ("String"=w231:string)  [unwired: 9 in, 1 out]
                n146 = Index Array(array=w229, index=3) -> (element=w230:cluster{string[]})
                n147 = property on="Ring" class="Ring (strict)"("Visible"=TRUE) -> ()  [unwired: 2 in, 2 out]
                n148 = property on="Slider" class="Slide (strict)"("Visible"=FALSE) -> ()  [unwired: 2 in, 2 out]
                n149 = Unbundle(w230) -> (w226:string[])
                n150 = Match First String(2:w226, 3:w231) -> (0:w227:i32)  [unwired: 1 out]
                n151 = property on="Ring" class="Ring (strict)"("Value"=w227, "Strings []"=w226) -> ()  [unwired: 2 in, 2 out]
              }
              frame "Color Enable  **" {
                n152 = call <vilib>:"NT Read String.vi"("Name"=w241) -> ("String"=w240:string)  [unwired: 9 in, 1 out]
                n153 = Index Array(array=w238, index=4) -> (element=w239:cluster{string[]})
                n154 = property on="Ring" class="Ring (strict)"("Visible"=TRUE) -> ()  [unwired: 2 in, 2 out]
                n155 = property on="Slider" class="Slide (strict)"("Visible"=FALSE) -> ()  [unwired: 2 in, 2 out]
                n156 = Unbundle(w239) -> (w235:string[])
                n157 = Match First String(2:w235, 3:w240) -> (0:w236:i32)  [unwired: 1 out]
                n158 = property on="Ring" class="Ring (strict)"("Value"=w236, "Strings []"=w235) -> ()  [unwired: 2 in, 2 out]
              }
              frame Default {
                n159 = property on="Slider" class="Slide (strict)"("Visible"=FALSE) -> ()  [unwired: 2 in, 2 out]
                n160 = property on="Ring" class="Ring (strict)"("Visible"=FALSE) -> ()  [unwired: 2 in, 2 out]
              }
              frame "Brightness  **", "Color Level  **", "Compression  **", "FPS  **", "Sharpness  **" {
                n161 = call <vilib>:"NT Read Number.vi"("Name"=w247) -> ("Numeric"=w246:dbl)  [unwired: 9 in, 1 out]
                n162 = property on="Ring" class="Ring (strict)"("Visible"=FALSE) -> ()  [unwired: 2 in, 2 out]
                n163 = property on="Slider" class="Slide (strict)"("Visible"=TRUE, "Scale.Maximum"=100.0 ("Scale.Range:Maximum")) -> ()  [unwired: 2 in, 2 out]
                n164 = local write "Slider"(w246) -> ()
              }
            }
            n165 = property on="Rev/Fwd" class="Clust (strict)"("Visible"=FALSE) -> ()  [unwired: 2 in, 2 out]
            n166 = property on="On/Off" class="Bool (strict)"("Visible"=FALSE) -> ()  [unwired: 2 in, 2 out]
          }
        }
      }
      event "Test Name": Mouse Enter {
        # "Populate the ring with the list of tests"
        n167 = event-data() -> ()  [unwired: 1 in, 1 out]
        n168 = call <vilib>:"NT Read String Array.vi"("Name"="TestMode/TestList") -> ("String Array"=w254:string[])  [unwired: 9 in, 1 out]
        n169 = Build Array (concatenate)("Select the test to run...", w254) -> (w253:string[])
        n170 = property on="Test Name" class="Ring (strict)"("Strings []"=w253) -> ()  [unwired: 2 in, 2 out]
      }
      event "Test Name": Value Change {
        w256 = FALSE ("Visible")
        # "Tell the robot the test name to run"
        n171 = event-data() -> ("NewVal"=w260:u16)  [unwired: 1 in]
        n172 = property on="Test Name" class="Ring (strict)"() -> ("Strings []"=w261:string[])  [unwired: 2 in, 2 out]
        n173 = property on="Ring" class="Ring (strict)"("Visible"=w256) -> ()  [unwired: 2 in, 2 out]
        n174 = property on="Motor" class="Clust (strict)"("Visible"=w256) -> ()  [unwired: 2 in, 2 out]
        n175 = property on="Slider" class="Slide (strict)"("Visible"=w256) -> ()  [unwired: 2 in, 2 out]
        n176 = property on="On/Off" class="Bool (strict)"("Visible"=w256) -> ()  [unwired: 2 in, 2 out]
        n177 = property on="Rev/Fwd" class="Clust (strict)"("Visible"=w256) -> ()  [unwired: 2 in, 2 out]
        n178 = local write "Progress"(T5 {"Test Progress"=0, "Test Progress Text"=""} ("Progress")) -> ()
        n179 = property on="Progress" class="Clust (strict)"("Visible"=TRUE) -> ()  [unwired: 2 in, 2 out]
        n180 = Index Array(array=w261, index=w260) -> (element=w259:string)
        n181 = call <vilib>:"NT Write String.vi"("String"=w259, "Name"="TestMode/TestName") -> ()  [unwired: 9 in, 1 out]
      }
      event "DB Camera Config": Value Change {
        n182 = event-data() -> ("NewVal"=w266:bool)  [unwired: 1 in]
        n183 = case shown="True" w266 {
          tunnel: w265 -> [w275 _]
          tunnel: [w268 w286] -> w264
          tunnel: w263 -> [w267 w286]
          frame False {
            w282 = "Camera"
            w285 = FALSE ("Visible")
            n184 = property on="Camera Settings" class="Clust (strict)"("Visible"=w285) -> ()  [unwired: 2 in, 2 out]
            n185 = local write "DB Camera Config"(w285) -> ()
            n186 = local read "Camera Settings"() -> (w274:T1)
            n187 = Index Array(array=w275) -> (element=w278:cluster{string[]})  [unwired: 1 in]
            n188 = Unbundle(w278) -> (w277:string[])
            n189 = Unbundle(w274) -> ("Frate Rate"=w273:i32, "Compression"=w272:i32, "Size"=w276:u16)
            n190 = Index Array(array=w277, index=w276) -> (element=w271:string)
            n191 = call-poly <vilib>:"Write Key.vi"("section"=w282, "value"=w271, "key"="Size", "refnum"=w267) -> ("refnum out"=w284:T7)  [unwired: 2 in, 5 out]
            n192 = call-poly <vilib>:"Write Key.vi"("section"=w282, "value"=w273, "key"="FrameRate", "refnum"=w284) -> ("refnum out"=w283:T7)  [unwired: 1 in, 6 out]
            n193 = call-poly <vilib>:"Write Key.vi"("section"=w282, "value"=w272, "key"="Compression", "refnum"=w283) -> ("refnum out"=w269:T7)  [unwired: 1 in, 6 out]
            n194 = call <vilib>:"Close Config Data.vi"("refnum"=w269) -> ("file path"=w270:path)  [unwired: 2 in, 8 out]
            n195 = call <vilib>:"Open Config Data.vi"("configuration file path"=w270) -> ("refnum"=w268:T7)  [unwired: 8 in, 2 out]
          }
          frame True {
            n196 = property on="Camera Settings" class="Clust (strict)"("Visible"=TRUE) -> ()  [unwired: 2 in, 2 out]
          }
        }
      }
      event "DB Camera Config 2": Value Change {
        n197 = event-data() -> ("NewVal"=w290:bool)  [unwired: 1 in]
        n198 = case shown="True" w290 {
          tunnel: [w294 w310] -> _
          tunnel: w289 -> [w293 _]
          tunnel: w288 -> [w292 w310]
          frame False {
            w307 = "Camera"
            w291 = FALSE ("Visible")
            n199 = local write "DB Camera Config 2"(w291) -> ()
            n200 = local read "Camera Settings 2"() -> (w300:T1)
            n201 = Index Array(array=w293) -> (element=w303:cluster{string[]})  [unwired: 1 in]
            n202 = property on="Camera Settings 2" class="Clust (strict)"("Visible"=w291) -> ()  [unwired: 2 in, 2 out]
            n203 = Unbundle(w303) -> (w302:string[])
            n204 = Unbundle(w300) -> ("Frate Rate"=w299:i32, "Compression"=w298:i32, "Size"=w301:u16)
            n205 = Index Array(array=w302, index=w301) -> (element=w297:string)
            n206 = call-poly <vilib>:"Write Key.vi"("section"=w307, "value"=w297, "key"="Size", "refnum"=w292) -> ("refnum out"=w309:T7)  [unwired: 2 in, 5 out]
            n207 = call-poly <vilib>:"Write Key.vi"("section"=w307, "value"=w299, "key"="FrameRate", "refnum"=w309) -> ("refnum out"=w308:T7)  [unwired: 1 in, 6 out]
            n208 = call-poly <vilib>:"Write Key.vi"("section"=w307, "value"=w298, "key"="Compression", "refnum"=w308) -> ("refnum out"=w295:T7)  [unwired: 1 in, 6 out]
            n209 = call <vilib>:"Close Config Data.vi"("refnum"=w295) -> ("file path"=w296:path)  [unwired: 2 in, 8 out]
            n210 = call <vilib>:"Open Config Data.vi"("configuration file path"=w296) -> ("refnum"=w294:T7)  [unwired: 8 in, 2 out]
          }
          frame True {
            n211 = property on="Camera Settings 2" class="Clust (strict)"("Visible"=TRUE) -> ()  [unwired: 2 in, 2 out]
          }
        }
      }
      event "Camera Settings": Value Change {
        n212 = event-data() -> ("NewVal"=w323:T1)  [unwired: 1 in]
        n213 = Index Array(array=w319) -> (element=w318:cluster{string[]})  [unwired: 1 in]
        n214 = Unbundle(w318) -> (w317:string[])
        n215 = Unbundle(w323) -> ("Frate Rate"=w314:i32, "Compression"=w313:i32, "Size"=w316:u16)
        n216 = Index Array(array=w317, index=w316) -> (element=w315:string)
        n217 = Format Into String(format string="%s   %dfps   %d%%", w315, w314, w313) -> (resulting string=w320:string)  [unwired: 2 in, 1 out]
        n218 = Build Array(w320) -> (w321:string[])
        n219 = property on="DB Camera Config" class="Bool (strict)"("Strings [4]"=w321) -> ()  [unwired: 2 in, 2 out]
      }
      event "Camera Settings 2": Value Change {
        n220 = event-data() -> ("NewVal"=w335:T1)  [unwired: 1 in]
        n221 = Index Array(array=w331) -> (element=w330:cluster{string[]})  [unwired: 1 in]
        n222 = Unbundle(w330) -> (w329:string[])
        n223 = Unbundle(w335) -> ("Frate Rate"=w326:i32, "Compression"=w325:i32, "Size"=w328:u16)
        n224 = Index Array(array=w329, index=w328) -> (element=w327:string)
        n225 = Format Into String(format string="%s   %dfps   %d%%", w327, w326, w325) -> (resulting string=w332:string)  [unwired: 2 in, 1 out]
        n226 = Build Array(w332) -> (w333:string[])
        n227 = property on="DB Camera Config 2" class="Bool (strict)"("Strings [4]"=w333) -> ()  [unwired: 2 in, 2 out]
      }
      event "Motor.Enable": Value Change {
        n228 = event-data() -> ("NewVal"=w341:bool)  [unwired: 1 in]
        n229 = Unbundle("Motor") -> ("Value"=w340:dbl)  [unwired: 1 out]
        n230 = Select(t=w340, s=w341, f=0.0) -> (s? t:f=w338:dbl)
        n231 = call <vilib>:"NT Write Number.vi"("Numeric"=w338, "Name"=w337) -> ()  [unwired: 9 in, 1 out]
      }
      event "Slider": Value Change {
        n232 = event-data() -> ("NewVal"=w344:dbl)  [unwired: 1 in]
        n233 = call <vilib>:"NT Write Number.vi"("Numeric"=w344, "Name"=w345) -> ()  [unwired: 9 in, 1 out]
      }
      event "On/Off": Value Change {
        n234 = event-data() -> ("NewVal"=w349:bool)  [unwired: 1 in]
        n235 = Boolean To (0,1)(Boolean=w349) -> (0, 1=w348:i16)
        n236 = call <vilib>:"NT Write Number.vi"("Numeric"=w348, "Name"=w347) -> ()  [unwired: 9 in, 1 out]
      }
      event "Rev/Fwd": Value Change {
        n237 = event-data() -> ("NewVal.Forward"=w357:bool, "NewVal.Reverse"=w356:bool)  [unwired: 1 in]
        n238 = Boolean To (0,1)(Boolean=w356) -> (0, 1=w355:i16)
        n239 = Boolean To (0,1)(Boolean=w357) -> (0, 1=w353:i16)
        n240 = Negate(x=w355) -> (-x=w354:i16)
        n241 = Add(x=w353, y=w354) -> (x+y=w352:i16)
        n242 = call <vilib>:"NT Write Number.vi"("Numeric"=w352, "Name"=w351) -> ()  [unwired: 9 in, 1 out]
      }
      event "Ring": Value Change {
        n243 = event-data() -> ("NewVal"=w361:u16)  [unwired: 1 in]
        n244 = property on="Ring" class="Ring (strict)"() -> ("Strings []"=w362:string[])  [unwired: 2 in, 2 out]
        n245 = Index Array(array=w362, index=w361) -> (element=w360:string)
        n246 = call <vilib>:"NT Write String.vi"("String"=w360, "Name"=w359) -> ()  [unwired: 9 in, 1 out]
      }
    }
  }
  n247 = property on="Camera Settings" class="Clust (strict)"("Val(Sgnl)"=w8) -> ()  [unwired: 2 in, 2 out]
  n248 = UDP Open(11:u16 1165 ("port")) -> (port=w43:refnum<k16>)  [unwired: 2 in, 4 out]
  n249 = while {
    tunnel: w43 -> [w369]
    tunnel: w34 -> [w364]
    tunnel: w30 -> [w367]
    tunnel: [w365] -> _
    i -> [w365]
    stop <- FALSE stop-if-true
    # "These subVIs decode errors, user data, game mode, etc.\nThey aren't connected to indicators by default"
    n250 = call "Receive DS Packet.vi"("Recv Socket"=w369) -> ("Battery"=→"Battery" →"Battery Value":sgl, "Robot IP Address"=w363:string, "Status"=w370:T8)  [unwired: 1 in, 11 out]
    "Robot IP" <- w363
    n251 = case shown="Default" w363 {
      selector: w363 -> [_ w380]
      tunnel: w364 -> [_ w381]
      frame "0.0.0.0" {
        # "Robot not responding, don't poll the variables"
      }
      frame Default {
        n252 = Send Notification(notification=w380, notifier=w381) -> ()  [unwired: 1 in, 2 out]
        n253 = call <vilib>:"SD Read Boolean.vi"("Name"="Manual Mode") -> ("Boolean"=→"Manual Mode":bool)  [unwired: 8 in, 2 out]
        n254 = call <vilib>:"SD Read Boolean.vi"("Name"="Climb Mode") -> ("Boolean"=→"Climb Mode":bool)  [unwired: 8 in, 2 out]
        n255 = call <vilib>:"SD Read Numeric Array.vi"("Name"="Joystick 2/Axes") -> ("Numeric Array"=w390:dbl[])  [unwired: 8 in, 2 out]
        n256 = call <vilib>:"SD Read Numeric Array.vi"("Name"="Joystick 1/Axes") -> ("Numeric Array"=w396:dbl[])  [unwired: 8 in, 2 out]
        n257 = call <vilib>:"SD Read Numeric Array.vi"("Name"="RobotDrive Motors") -> ("Numeric Array"=w402:dbl[])  [unwired: 8 in, 2 out]
        n258 = call <vilib>:"SD Read Boolean Array.vi"("Name"="Joystick 1/Buttons") -> ("Boolean Array"=w397:bool[])  [unwired: 8 in, 2 out]
        n259 = call <vilib>:"SD Read Boolean Array.vi"("Name"="Joystick 2/Buttons") -> ("Boolean Array"=w389:bool[])  [unwired: 8 in, 2 out]
        n260 = Index Array(array=w390) -> (element #1=w385:dbl, element #2=w384:dbl, element #3=→"JS2 Z":dbl)  [unwired: 3 in]
        n261 = Index Array(array=w396) -> (element #1=w393:dbl, element #2=w394:dbl, element #3=→"JS1 Z":dbl)  [unwired: 6 in, 3 out]
        n262 = Index Array(array=w402) -> (element #1=→"MotorChart1" →"MotorSlide1":dbl, element #2=→"MotorSlide2" →"MotorChart2":dbl, element #3=→"MotorChart3" →"MotorSlide3":dbl, element #4=→"MotorChart4" →"MotorSlide4":dbl)  [unwired: 4 in]
        n263 = Array To Cluster(array=w397) -> (cluster=w378:T9)
        "JS Buttons 1" <- w378
        n264 = Array To Cluster(array=w389) -> (cluster=w379:T9)
        "JS Buttons 2" <- w379
        n265 = Unbundle By Name(w378) -> ("Boolean Array[0]"=→"Driver Ready":bool)
        n266 = Unbundle By Name(w379) -> ("Boolean Array[0]"=→"Shooter Ready":bool)
        n267 = Bundle("Numeric"=w385, "Numeric"=w384) -> (w386:cluster{"Numeric":dbl, "Numeric":dbl})  [unwired: 1 in]
        n268 = Bundle("Numeric"=w393, "Numeric"=w394) -> (w392:cluster{"Numeric":dbl, "Numeric":dbl})  [unwired: 1 in]
        n269 = Build Array(w386) -> (→"Joystick 2":cluster{"Numeric":dbl, "Numeric":dbl}[])
        n270 = Build Array(w392) -> (→"Joystick 1":cluster{"Numeric":dbl, "Numeric":dbl}[])
      }
    }
    n271 = call "Decode Status Byte.vi"("Window Mode Notifier"=w367, "Status"=w370) -> ("Mode"=→"Mode":T3)  [unwired: 1 out]
  }
  n272 = while {
    tunnel: w30 -> [w424]
    tunnel: [w422] -> _
    i -> [w422]
    stop <- FALSE stop-if-true
    w414 = 1300  # width
    w417 = 400  # height
    # "If DS is docked, like when\nlogged in as Driver, place just\nabove DS, otherwise, move\ntitlebar onscreen. Show or hide\ntitlebar and other attributes to match\nDS."
    n273 = Wait on Notification(notifier=w424) -> (notification=w409:bool)  [unwired: 3 in, 3 out]
    n274 = property class="App"() -> ("Disp.WkSpace"=w420:T10)  [unwired: 2 in, 2 out]
    n275 = Not(x=w409) -> (.not. x?=w423:bool)
    n276 = Select(t=0, s=w409, f=30) -> (s? t:f=w408:i32)
    n277 = Unbundle(w420) -> ("Left"=w418:i16, "Bottom"=w415:i16)  [unwired: 2 out]
    n278 = property class="VI"("Front Panel.Closeable"=w423, "Front Panel.Minimizeable"=w423, "Front Panel.TitleBarVis"=w423) -> ()  [unwired: 2 in, 2 out]
    n279 = Subtract(x=w415, y=600) -> (x-y=w412:i32)
    n280 = Add(x=w418, y=w414) -> (x+y=w419:i32)
    n281 = In Range and Coerce(upper limit=100000, x=w412, lower limit=w408) -> (coerced(x)=w406:i32)  [unwired: 1 out]
    n282 = Add(x=w406, y=w417) -> (x+y=w416:i32)
    n283 = Bundle("Left"=w418, w406, w419, w416) -> (w421:cluster{"Left":i16, i32, i32, i32})  [unwired: 1 out]
    n284 = property class="VI"("Front Panel.PanelBounds"=w421) -> ()  [unwired: 2 in, 2 out]
  }
